vi "type.get.vi"(8 "error in":errorcluster, 10 "Type RID":string, 11 "Nominal Client in":refnum<class "Nominal Client.lvclass">) -> (0 "error out":errorcluster, 2 "type":refnum<class "type.lvclass">, 3 "Nominal Client out":refnum<class "Nominal Client.lvclass">)   [LabVIEW 2020, in "Nominal Client.lvclass"]
uses:
  Nominal Client.lvclass
  type/type.lvclass
  50f5c392-d963-4889-9ba8-5574e989f4eb.vi
  <vilib>/JDP Science/JSONtext/Variant to JSON Text.vi
  <vilib>/JDP Science/JSONtext/LVClass Serializer/JSONtext LVClass Serializer.lvclass
  <vilib>/JDP Science/JSONtext/JSONtext.lvlib
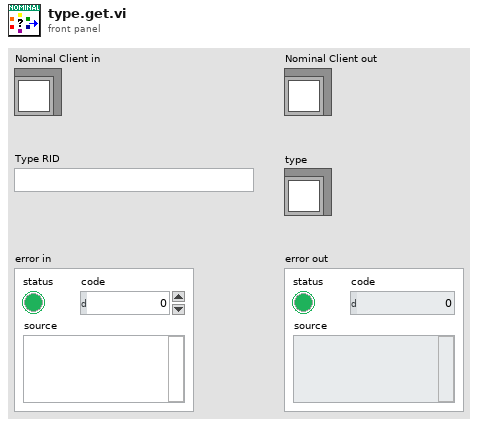
[diagram p1: front panel]
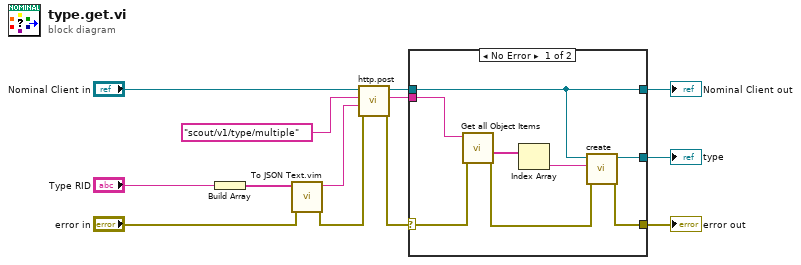
[diagram p0: block diagram]
diagram:
  n1 = Build Array("Type RID") -> (w7:string[])
  n2 = call "To JSON Text.vim"("error in (no error)"="error in", "Anything"=w7) -> ("error out"=w8:errorcluster, "<JSON>"=w9:string)  [unwired: 8 in]
  n3 = call "http.post.vi"("error in"=w8, "Request body"=w9, "Path"="scout/v1/type/multiple", "Nominal Client in"="Nominal Client in") -> ("error out"=w11:errorcluster, "Response"=w13:string, "Nominal Client out"=w12:refnum<class "Nominal Client.lvclass">)  [unwired: 5 in]
  n4 = case shown="No Error" w11 {
    selector: w11 -> [w19 w23]
    tunnel: w13 -> [w21 _]
    tunnel: w12 -> [w18 w22]
    tunnel: [w18 w22] -> w5
    tunnel: [w15 w23] -> w2
    tunnel: [w14 _] -> w4
    frame No Error {
      n5 = call <vilib>:"Get all Object Items.vi"("error in (no error)"=w19, "JSON"=w21) -> ("error out"=w16:errorcluster, "<JSON>"=w20:string[])  [unwired: 6 in, 2 out]
      n6 = Index Array(array=w20) -> (element=w17:string)  [unwired: 1 in]
      n7 = call "create.vi"("error in"=w16, "type"=w17, "Nominal Client"=w18) -> ("error out"=w15:errorcluster, "type"=w14:refnum<class "type.lvclass">)  [unwired: 7 in]
    }
    frame Error {
    }
  }
  "Nominal Client out" <- w5
  "error out" <- w2
  "type" <- w4
